vi "Write.vi"(8 "error in (no error)":errorcluster, 9 "write enable":bool=TRUE, 11 "ICPCON ET7024 in":refnum<class "ICPCON ET-7024.lvclass">) -> (0 "error out":errorcluster, 3 "ICPCON ET7024 out":refnum<class "ICPCON ET-7024.lvclass">)   [LabVIEW 2021, in "ICPCON ET-7024.lvclass"]
uses:
  ICPCON ET-7024.lvclass
  D:/my_projects/projects/Algorithms/Labview/21/Master CR/Master CR.lvclass
  D:/my_projects/projects/Algorithms/Labview/21/Master CR/Devices/ET7000/TCP/TCP.lvclass
  Master CR.lvclass/Master CR.ctl
  Modbus_v121c/Modbus Data Unit/Modbus Data Unit.lvclass/Modbus Data Unit.ctl
  Modbus_v121c/Network Protocol/Network Master/Network Master.lvclass/Network Master.ctl
  Modbus_v121c/Master Function Definition/Write Multiple Registers Request.vi
  Modbus_v121c/Master Function Definition/Function data mismatch error.vi
  Modbus_v121c/Master Function Definition/Write Multiple Registers Response.vi
  Modbus_v121c/Network Protocol/Network Master/Read write Master.vi
  Modbus_v121c/Master Function Definition/Read Holding Registers Request.vi
  Modbus_v121c/Master Function Definition/Read Holding Registers Response.vi
  Modbus_v121c/Master Function Definition/Write Multiple Coils Request.vi
  Modbus_v121c/Master Function Definition/Write Multiple Coils Response.vi
  Modbus_v121c/Master Function Definition/Read Coils Request.vi
  Modbus_v121c/Master Function Definition/Read Coils Response.vi
  Network Protocol/Read Network Protocol.vi
  Modbus_v121c/Modbus Data Unit/Construct PDU.vi
  Modbus_v121c/Utility/U16s to Bytes.vi
  Modbus_v121c/Master Function Definition/Function code mismatch error.vi
  Modbus_v121c/Data Model/Error Generator.vi
  Modbus_v121c/Modbus Data Unit/Deconstruct PDU.vi
  Modbus_v121c/Utility/Bytes to U16s.vi
  Modbus_v121c/Utility/Bits to Bytes.vi
  Modbus_v121c/Utility/Bytes to Bits.vi
  TCP/TCP.lvclass
  Modbus_v121c/Network Protocol/Network Master/Network Master.lvclass
  Modbus_v121c/Modbus Data Unit/Modbus Data Unit.lvclass
  Modbus_v121c/Data Model/Device Data Model.lvclass
  Modbus_v121c/Transmission Data Unit/Transmission Data Unit.lvclass
  Master CR.lvclass
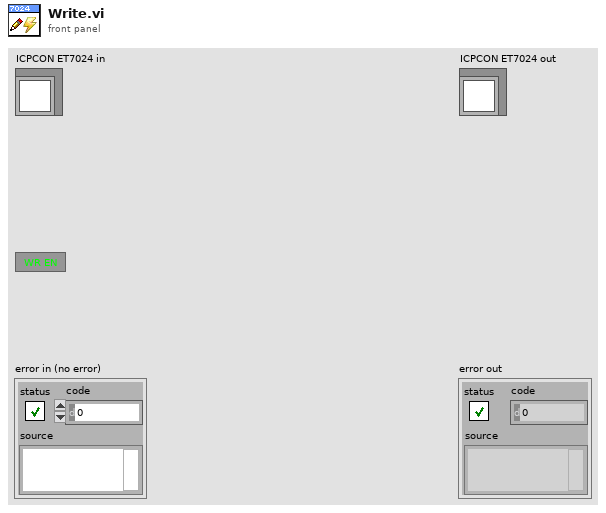
[diagram p1: front panel]
types:
  T1 = typedef "Device Data Model.lvclass/N channel.ctl" = cluster{"N DI channel":i32, "N DO channel":i32, "N AI channel":i32, "N AO channel":i32}
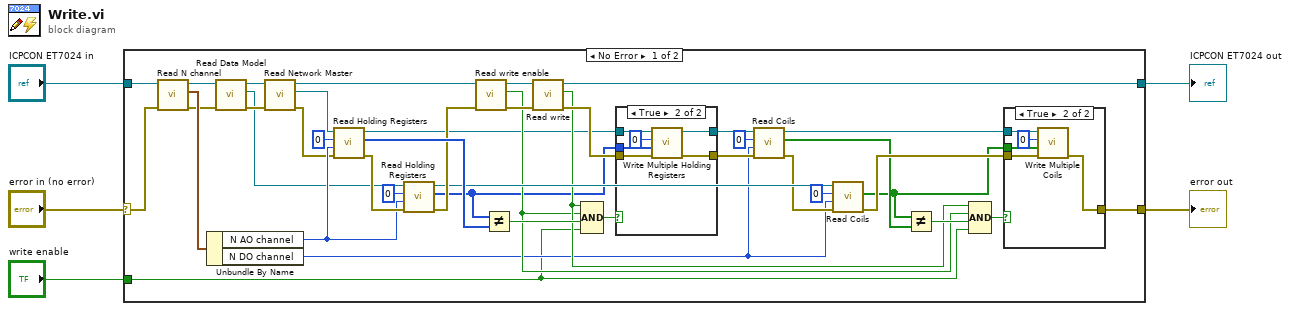
[diagram p0: block diagram]
diagram:
  n1 = case shown="No Error" "error in (no error)" {
    selector: "error in (no error)" -> [w43 w63]
    tunnel: [w16 w63] -> w3
    tunnel: [w13 w62] -> w4
    tunnel: "ICPCON ET7024 in" -> [w45 w62]
    tunnel: "write enable" -> [w17 _]
    frame No Error {
      n2 = call "Read N channel.vi"("error in (no error)"=w43, "Master CR in"=w45) -> ("error out"=w42:errorcluster, "N channel"=w46:T1, "Master CR out"=w44:refnum<class "ICPCON ET-7024.lvclass">)  [unwired: 7 in]
      n3 = Unbundle By Name(w46) -> ("N AO channel"=w32:i32, "N DO channel"=w19:i32)
      n4 = call "Read Data Model.vi"("error in (no error)"=w42, "Master CR in"=w44) -> ("error out"=w11:errorcluster, "Data Model"=w7:refnum<class "Device Data Model.lvclass">, "Master CR out"=w12:refnum<class "ICPCON ET-7024.lvclass">)  [unwired: 7 in]
      n5 = call "Read Network Master.vi"("error in (no error)"=w11, "TCP in"=w12) -> ("error out"=w6:errorcluster, "Network Master"=w8:refnum<class "Network Master.lvclass">, "TCP out"=w9:refnum<class "ICPCON ET-7024.lvclass">)  [unwired: 7 in]
      n6 = call "Read Holding Registers.vi"("error in (no error)"=w6, "number of holding registers"=w32, "starting address"=u16 0, "Modbus master in"=w8) -> ("error out"=w33:errorcluster, "register values"=w35:u16[], "Modbus master out"=w10:refnum<class "Network Master.lvclass">)  [unwired: 5 in]
      n7 = call-dynamic "Read Holding Registers.vi"("error in"=w33, "number of registers"=w32, "starting address"=u16 0, "device data model in"=w7) -> ("error out"=w34:errorcluster, "data"=w15:u16[], "device data model out"=w29:refnum<class "Device Data Model.lvclass">)  [unwired: 5 in]
      n8 = call "Read write enable.vi"("error in (no error)"=w34, "Master CR in"=w9) -> ("error out"=w39:errorcluster, "write enable"=w26:bool, "Master CR out"=w40:refnum<class "ICPCON ET-7024.lvclass">)  [unwired: 7 in]
      n9 = Not Equal?(x=w15, y=w35) -> (x != y?=w41:bool)
      n10 = call "Read write.vi"("error in (no error)"=w39, "Master CR in"=w40) -> ("error out"=w38:errorcluster, "Write"=w27:bool, "Master CR out"=w13:refnum<class "ICPCON ET-7024.lvclass">)  [unwired: 7 in]
      n11 = Compound Arithmetic op=AND(w27, w26, w41, w17) -> (w47:bool)
      n12 = case shown="True" w47 {
        tunnel: w38 -> [w49 w54]
        tunnel: [w49 w52] -> w20
        tunnel: w15 -> [_ w53]
        tunnel: [w48 w51] -> w21
        tunnel: w10 -> [w48 w50]
        frame False {
        }
        frame True {
          n13 = call "Write Multiple Holding Registers.vi"("error in (no error)"=w54, "holding register values"=w53, "starting address"=u16 0, "Modbus master in"=w50) -> ("error out"=w52:errorcluster, "Modbus master out"=w51:refnum<class "Network Master.lvclass">)  [unwired: 6 in]
        }
      }
      n14 = call "Read Coils.vi"("error in (no error)"=w20, "number of coils"=w19, "starting address"=u16 0, "Modbus master in"=w21) -> ("error out"=w23:errorcluster, "coil values"=w24:bool[], "Modbus master out"=w25:refnum<class "Network Master.lvclass">)  [unwired: 5 in]
      n15 = call-dynamic "Read Coils.vi"("error in"=w23, "number of coils"=w19, "starting address"=u16 0, "device data model in"=w29) -> ("error out"=w28:errorcluster, "data"=w14:bool[])  [unwired: 5 in, 1 out]
      n16 = Not Equal?(x=w14, y=w24) -> (x != y?=w31:bool)
      n17 = Compound Arithmetic op=AND(w27, w26, w31, w17) -> (w30:bool)
      n18 = case shown="True" w30 {
        tunnel: w28 -> [w56 w60]
        tunnel: [w56 w57] -> w16
        tunnel: w14 -> [_ w59]
        tunnel: w25 -> [_ w61]
        frame False {
        }
        frame True {
          n19 = call "Write Multiple Coils.vi"("error in (no error)"=w60, "coil values"=w59, "starting address"=u16 0, "Modbus master in"=w61) -> ("error out"=w57:errorcluster)  [unwired: 6 in, 1 out]
        }
      }
    }
    frame Error {
    }
  }
  "error out" <- w3
  "ICPCON ET7024 out" <- w4
